vi "Wake HL.vi"(7 "VISA resource":refnum<visa-resource-name>, 8 "error in":errorcluster, 9 "Timeout":i32, 10 "Comando":T1 {"Step style motor 2" items=["Medio paso", "Paso completo"]; "Step style motor 1" items=["Medio paso", "Paso completo"]; "Direction motor 2" items=["", "Forward", "Backward"]; "Direction motor 1" items=["", "Forward", "Backward"]; "Action" items=["Initialize", "Move"]}, 11 "Module ID":i32=-1) -> (0 "error out":errorcluster)   [LabVIEW 2020, in "Arduino-Adafruit stepper.lvlib"]
doc: "<b>Note</b>: This VI was renamed by the DQMH Rename Event utility. Make sure the VI Description is updated to reflect the new event name, then delete this comment.\n\nRequest to start moving motors.\n_____\nCreated using DQMH Event Scripter 7.0.1.1316."
uses:
  Arduino-Adafruit stepper.lvlib
  Arduino stepper library/Public/Controls/Move motor parameters--cluster.ctl
  Arduino stepper library/Public/Controls/Motor direction.ctl
  Arduino stepper library/Public/Controls/Step style.ctl
  Wake HL Argument--cluster.ctl
  Arduino stepper library/Control de MaP.lvlib
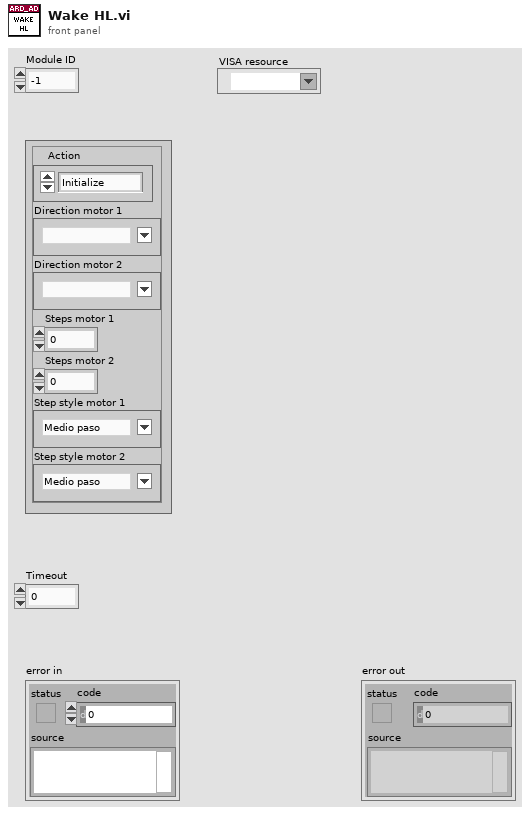
[diagram p1: front panel]
types:
  T1 = typedef "Control de MaP.lvlib/Move motor parameters--cluster.ctl" = cluster{"Action":u8, "Direction motor 1":T2, "Direction motor 2":T2, "Steps motor 1":u16, "Steps motor 2":u16, "Step style motor 1":T3, "Step style motor 2":T3}
  T2 = typedef "Control de MaP.lvlib/Motor direction.ctl" = u8
  T3 = typedef "Control de MaP.lvlib/Step style.ctl" = u8
  T4 = typedef "Arduino-Adafruit stepper.lvlib/Wake HL Argument--cluster.ctl" = cluster{"Module ID":i32, "Comando":T1, "Timeout":i32, "VISA resource":refnum<visa-resource-name>}
  T5 = typedef "Arduino-Adafruit stepper.lvlib/Request Events--cluster.ctl" = cluster{"Stop Module":refnum<user-event>, "Show Panel":refnum<user-event>, "Hide Panel":refnum<user-event>, "Show Diagram":refnum<user-event>, "Get Module Execution Status":refnum<user-event>, "Initialize Arduino":refnum<user-event>, "Connect":refnum<user-event>, "Disconnect":refnum<user-event>, "Init motors":refnum<user-event>, "Home motors":refnum<user-event>, "Begin movement":refnum<user-event>, "Wake HL":refnum<user-event>, "Stop movement":refnum<user-event>, "Sleep HL":refnum<user-event>}
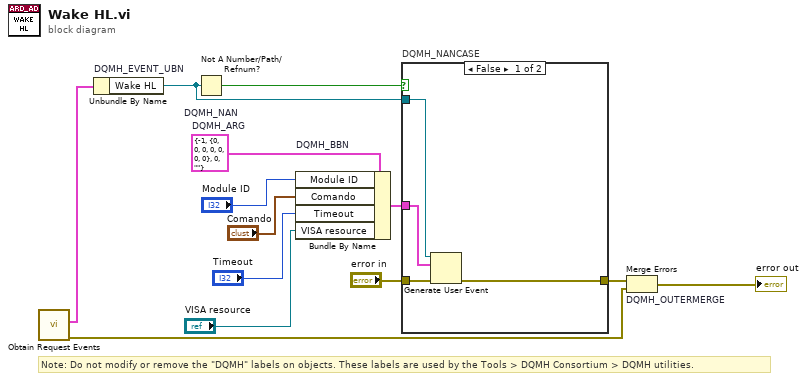
[diagram p0: block diagram]
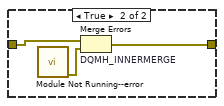
[diagram p2: hidden frame]
diagram:
  w7 = T4 {"Module ID"=-1, "Comando"={"Action"=0, "Direction motor 1"=0, "Direction motor 2"=0, "Steps motor 1"=0, "Steps motor 2"=0, "Step style motor 1"=0, "Step style motor 2"=0}, "Timeout"=0, "VISA resource"=""}  # DQMH_ARG
  # "Note: Do not modify or remove the \"DQMH\" labels on objects. These labels are used by the Tools > DQMH Consortium > DQMH utilities."
  n1 = call "Obtain Request Events.vi"() -> ("error out"=w2:errorcluster, "Arduino-Adafruit stepper Request Events"=w1:T5)  [unwired: 10 in]
  n2 = Unbundle By Name "DQMH_EVENT_UBN"(w1) -> ("Wake HL"=w9:refnum<user-event>)
  n3 = Not A Number/Path/Refnum? "DQMH_NAN"(number/path/refnum=w9) -> (NaN/Path/Refnum?=w10:bool)
  n4 = Bundle By Name "DQMH_BBN"(cluster=w7, "Module ID"="Module ID", "Comando"="Comando", "Timeout"="Timeout", "VISA resource"="VISA resource") -> (w11:T4)
  n5 = case "DQMH_NANCASE" shown="False" w10 {
    tunnel: "error in" -> [w17 w20]
    tunnel: [w16 w19] -> w8
    tunnel: w9 -> [w15 _]
    tunnel: w11 -> [w14 _]
    frame False {
      n6 = Generate User Event(user event=w15, event data cluster=w14, error in=w17) -> (error out=w16:errorcluster)  [unwired: 1 in, 1 out]
    }
    frame True {
      n7 = call "Module Not Running--error.vi"() -> ("error out"=w18:errorcluster)  [unwired: 11 in]
      n8 = Merge Errors "DQMH_INNERMERGE"(w20, w18) -> (w19:errorcluster)
    }
  }
  n9 = Merge Errors "DQMH_OUTERMERGE"(w8, w2) -> (→"error out":errorcluster)
